vi "Catch Process Error.vi"(10 "Process Error":errorcluster, 11 "SMO":refnum<class "SMO.lvclass">) -> (0 "error out":errorcluster, 3 "SMO out":refnum<class "SMO.lvclass">)   [LabVIEW 2013, in "SMO.lvclass"]
uses:
  SMO.lvclass
  SMO.lvclass/SMO.ctl
panel:
  # "For instructions on how to use the JKI State Machine Objects, examples and video tutorials, visit:\nhttp://jki.net/state-machine-objects/\n\nJKI State Machine Objects™\nhttp://jki.net/state-machine-objects/\nCopyright (C) 2005-2015, JKI <info@jki.net>\nALL RIGHTS RESERVED"
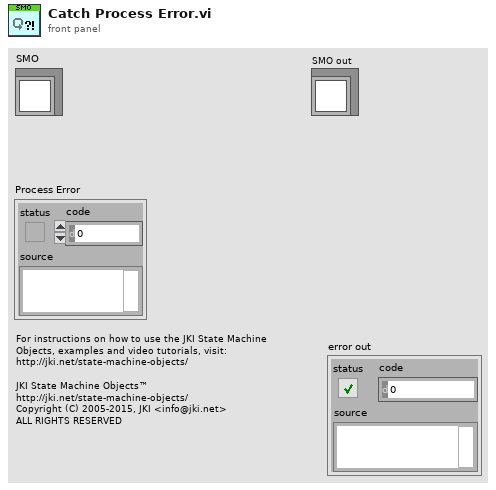
[diagram p1: front panel]
types:
  T1 = typedef "SMO.lvclass/PrivateData--Ref.ctl" = refnum<data-value>
  T2 = typedef "SMO.lvclass/PrivateData--Cluster.ctl" = cluster{"Parent Call":T3, "Registered Processes":T4[], "Sync Notifier":refnum<notifier>, "Process Error Notifier":refnum<notifier>, "Protected Events":T5, "Public Events":T6, "SMO State":T7, "[Dependencies]":T8[], "[Attributes]":refnum<class "Attribute.lvclass">[], "Launcher Close":refnum<notifier>, "Caller Watchdog":refnum<queue>, "Accessibility":T9}
  T3 = typedef "SMO.lvclass/Parent Call--Enum.ctl" = enum16{"Allows parent to run", "Does not request parent to run"}
  T4 = typedef "SMO.lvclass/RegisteredProcessData--Cluster.ctl" = cluster{"Name":string, "Static VI Ref":refnum<vi>, "Running":bool, "NotifierRef":u32}
  T5 = typedef "SMO.lvclass/Protected Events.ctl" = cluster{"StopProcesses":refnum<user-event>, "AbortProcesses":refnum<user-event>, "Config Changed":refnum<user-event>, "Dependency":refnum<user-event>}
  T6 = typedef "SMO.lvclass/Public Events.ctl" = cluster{"Error":refnum<user-event>, "State":refnum<user-event>, "Reserve State":refnum<user-event>}
  T7 = typedef "SMO.lvclass/SMOState --Enum.ctl" = enum16{"unknown", "Created", "Started", "Stopped"}
  T8 = typedef "SMO.lvclass/SMO Dependency--Cluster.ctl" = cluster{"Dependency":refnum<class "SMO.lvclass">, "Level":string}
  T9 = typedef "SMO.lvclass/Accessibility--Cluster.ctl" = cluster{"Lock Key":string, "Reserve State":T10}
  T10 = typedef "SMO.lvclass/Reserve State--Enum.ctl" = enum16{"Unreserved", "Reserved", "Self-locked"}
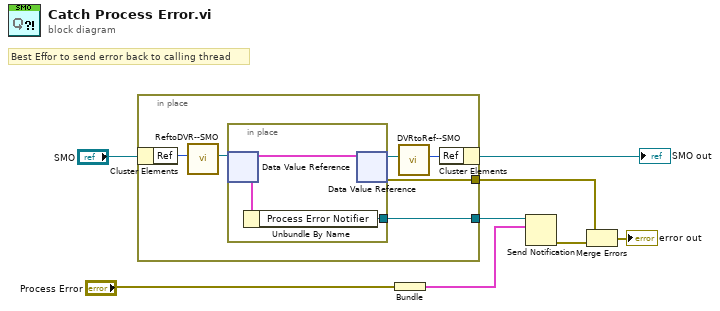
[diagram p0: block diagram]
diagram:
  # "Best Effor to send error back to calling thread"
  n1 = in-place {
    in-place-border: [w14] -> w7
    in-place-border: [w13] -> w3
    n2 = in-place-cluster #1("SMO") -> ("Ref"=w12:u32)
    n3 = call "ReftoDVR--SMO.vi"("Ref"=w12) -> ("Ref"=w11:T1)  [unwired: 10 in]
    n4 = in-place {
      in-place-border: [w16] -> w14
      n5 = in-place-dvr #2(w11) -> (w15:T2)  [unwired: 1 out]
      n6 = Unbundle By Name(w15) -> ("Process Error Notifier"=w16:refnum<notifier>)
      n7 = in-place-dvr #2(w15) -> (w10:T1, w13:errorcluster)
    }
    n8 = call "DVRtoRef--SMO.vi"("Ref"=w10) -> ("Ref"=w9:u32)  [unwired: 10 in]
    n9 = in-place-cluster #1("Ref"=w9) -> (→"SMO out":refnum<class "SMO.lvclass">)
  }
  n10 = Bundle("Process Error"="Process Error") -> (w5:cluster{"Process Error":errorcluster})  [unwired: 1 in]
  n11 = Send Notification(notification=w5, notifier=w7) -> (error out=w4:errorcluster)  [unwired: 1 in, 1 out]
  n12 = Merge Errors(w3, w4) -> (→"error out":errorcluster)
